vi "sub_SDR_mod_BPSK2QAM16.vi"(11 "Array in":i16[](array[numeric])) -> (3 "Array out":cdb[](array[numeric]))   [LabVIEW 2012]
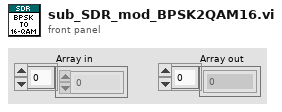
[diagram p1: front panel]
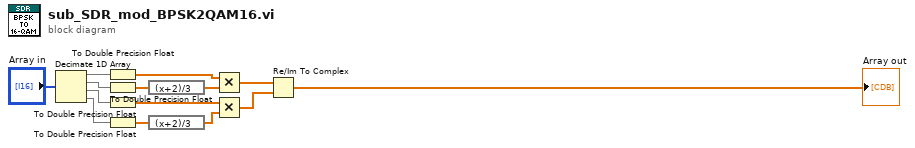
[diagram p0: block diagram]
diagram:
  n1 = Decimate 1D Array("Array in") -> (w6:i16[], w7:i16[], w8:i16[], w9:i16[])
  n2 = To Double Precision Float(number=w6) -> (double precision float=w11:dbl[])
  n3 = To Double Precision Float(number=w7) -> (double precision float=w4:dbl[])
  n4 = To Double Precision Float(number=w8) -> (double precision float=w14:dbl[])
  n5 = To Double Precision Float(number=w9) -> (double precision float=w3:dbl[])
  n6 = expression code="(x+2)/3"(w4) -> (w12:dbl[])
  n7 = expression code="(x+2)/3"(w3) -> (w13:dbl[])
  n8 = Multiply(x=w11, y=w12) -> (x*y=w2:dbl[])
  n9 = Multiply(x=w14, y=w13) -> (x*y=w1:dbl[])
  n10 = Re/Im To Complex(1:w1, 2:w2) -> (0:→"Array out":cdb[])
